vi "Align N Waveforms (continuous).vi"(4 "interpolation":bool=TRUE, 6 "FIR filter specifications":T1={"alias rejection (dB)"=120.0, "normalized bandwidth"=0.4536} {"normalized bandwidth" format="%.4f"; "alias rejection (dB)" format="%.2f"}, 7 "reset":bool, 8 "error in (no error)":errorcluster, 9 "interpolation mode":u16(ring)=1 items=["coerce", "linear", "spline", "FIR filter"], 11 "waveforms in":waveform(dbl)[](array[waveform])) -> (0 "error out":errorcluster, 3 "waveforms out":waveform(dbl)[](array[waveform]))   [LabVIEW 2020, in "NI_MAPro.lvlib"]
doc: "Performs element-wise alignment of waveforms and returns the aligned waveforms. The data types you wire to the waveform inputs determine the polymorphic instance to use."
uses:
  NI_MAPro.lvlib
  NI_MABase.lvlib
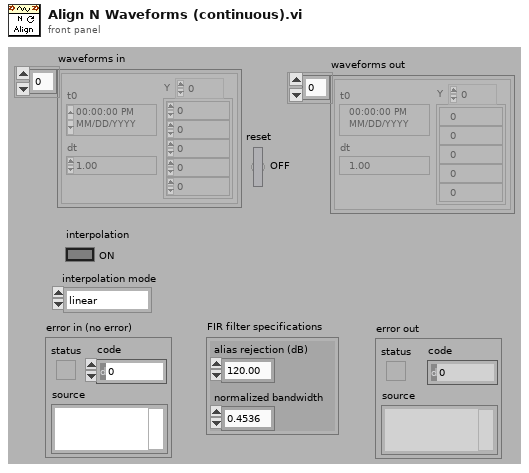
[diagram p1: front panel]
types:
  T1 = cluster{"alias rejection (dB)":dbl, "normalized bandwidth":dbl}
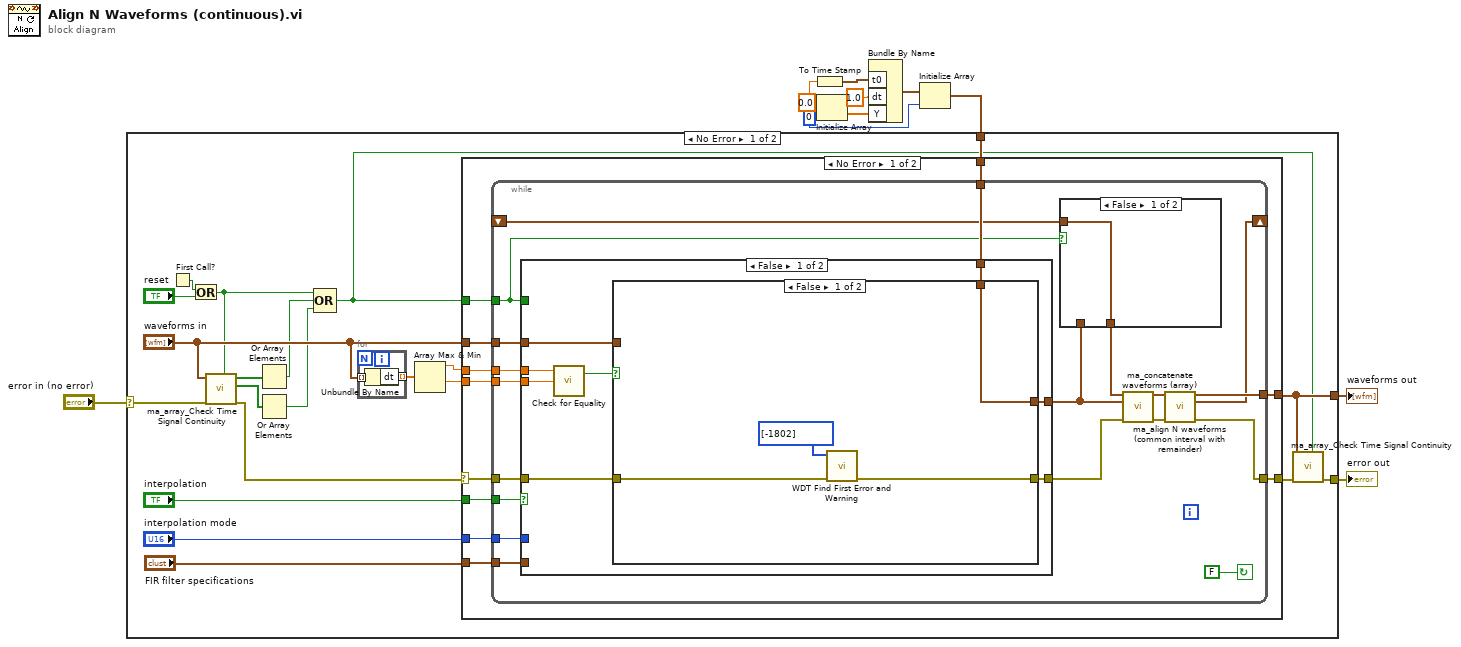
[diagram p0: block diagram]
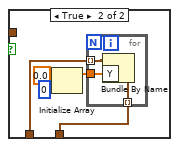
[diagram p2: hidden frame]
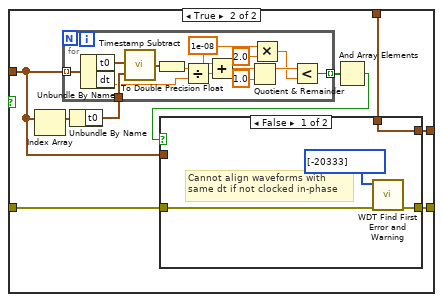
[diagram p3: hidden frame]
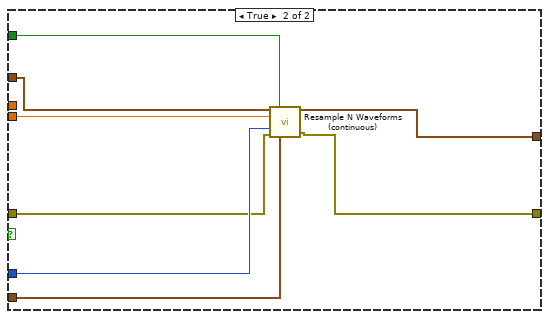
[diagram p5: hidden frame]
diagram:
  w4 = 0 ("dimension size")
  w7 = 0.0 ("element")
  n1 = To Time Stamp(1:w7) -> (0:w1:timestamp)
  n2 = Initialize Array(w7, w4) -> (w8:dbl[])
  n3 = Bundle By Name("t0"=w1, "dt"=1.0 ("element"), "Y"=w8) -> (w5:waveform(dbl))  [unwired: 1 in]
  n4 = Initialize Array(w5, w4) -> (w3:waveform(dbl)[])
  n5 = case shown="No Error" "error in (no error)" {
    selector: "error in (no error)" -> [w29 w125]
    tunnel: [w20 w125] -> w10
    tunnel: [w18 w124] -> w9
    tunnel: w3 -> [w25 w124]
    frame No Error {
      n6 = First Call?() -> (First Call?: T/F=w27:bool)
      n7 = Or(x=w27, y="reset") -> (x .or. y?=w17:bool)
      n8 = call "ma_array_Check Time Signal Continuity.vi"("Ignore input time stamp"=w17, "error in (no error)"=w29, "waveforms"="waveforms in") -> ("error out"=w14:errorcluster, "dt changed"=w13:bool[], "t0 changed"=w15:bool[])  [unwired: 5 in, 1 out]
      n9 = Or Array Elements(Boolean array=w15) -> (logical OR=w12:bool)
      n10 = Or Array Elements(Boolean array=w13) -> (logical OR=w11:bool)
      n11 = Compound Arithmetic op=OR(w17, w12, w11) -> (w16:bool)
      n12 = for {
        tunnel: "waveforms in" -> [w33] mode=indexing
        tunnel: [w32] -> w23 mode=indexing
        n13 = Unbundle By Name(w33) -> ("dt"=w32:dbl)
      }
      n14 = Array Max & Min(array=w23) -> (max value=w22:dbl, min value=w21:dbl)  [unwired: 2 out]
      n15 = case shown="No Error" w14 {
        selector: w14 -> [w39 w123]
        tunnel: "waveforms in" -> [w44 _]
        tunnel: w22 -> [w43 _]
        tunnel: w21 -> [w42 _]
        tunnel: [w38 w123] -> w19
        tunnel: [w41 w122] -> w18
        tunnel: w25 -> [w40 w122]
        tunnel: "interpolation mode" -> [w37 _]
        tunnel: "interpolation" -> [w36 _]
        tunnel: w16 -> [w35 _]
        tunnel: "FIR filter specifications" -> [w34 _]
        frame No Error {
          n16 = while {
            tunnel: w44 -> [w63]
            tunnel: w43 -> [w62]
            tunnel: w42 -> [w61]
            tunnel: [w53] -> w41
            tunnel: w40 -> [w60]
            tunnel: w39 -> [w59]
            tunnel: [w50] -> w38
            tunnel: w37 -> [w58]
            tunnel: w36 -> [w57]
            tunnel: w35 -> [w55]
            shift-right: [w47] -> _
            shift-left: _ -> [w45]
            tunnel: w34 -> [w48]
            stop <- FALSE continue-if-true
            n17 = case shown="False" w57 {
              tunnel: w63 -> [w80 w120]
              tunnel: w62 -> [w79 _]
              tunnel: w61 -> [w78 w118]
              tunnel: w60 -> [w76 _]
              tunnel: w59 -> [w75 w114]
              tunnel: [w74 w117] -> w52
              tunnel: w58 -> [_ w116]
              tunnel: w55 -> [_ w119]
              tunnel: w48 -> [_ w115]
              tunnel: [w73 w121] -> w46
              frame False {
                n18 = call "Check for Equality.vi"("n2"=w78, "n1"=w79) -> ("equal?"=w77:bool)  [unwired: 1 in, 1 out]
                n19 = case shown="False" w77 {
                  tunnel: w80 -> [_ w88]
                  tunnel: w76 -> [w81 w93]
                  tunnel: w75 -> [w84 w91]
                  tunnel: [w83 w92] -> w74
                  tunnel: [w81 w89] -> w73
                  frame False {
                    n20 = call "WDT Find First Error and Warning.vi"("error in (no error)"=w84, "Error Codes"=i32[] [-1802]) -> ("error out"=w83:errorcluster)  [unwired: 4 in, 1 out]
                  }
                  frame True {
                    n21 = Index Array(array=w88) -> (element=w87:waveform(dbl))  [unwired: 1 in]
                    n22 = Unbundle By Name(w87) -> ("t0"=w85:timestamp)
                    n23 = for {
                      tunnel: w88 -> [w107] mode=indexing
                      tunnel: w85 -> [w106]
                      tunnel: [w102] -> w90 mode=indexing
                      w99 = 1e-08
                      n24 = Unbundle By Name(w107) -> ("t0"=w96:timestamp, "dt"=w103:dbl)
                      n25 = call "Timestamp Subtract.vi"("y"=w106, "x"=w96) -> ("x - y"=w95:timestamp)
                      n26 = To Double Precision Float(number=w95) -> (double precision float=w94:dbl)
                      n27 = Divide(x=w94, y=w103) -> (x/y=w101:dbl)
                      n28 = Add(x=w99, y=w101) -> (x+y=w100:dbl)
                      n29 = Quotient & Remainder(x=w100, y=1.0) -> (x-y*floor(x/y)=w104:dbl)  [unwired: 1 out]
                      n30 = Multiply(x=w99, y=2.0) -> (x*y=w97:dbl)
                      n31 = Less?(x=w104, y=w97) -> (x < y?=w102:bool)
                    }
                    n32 = And Array Elements(Boolean array=w90) -> (logical AND=w86:bool)
                    n33 = case shown="False" w86 {
                      tunnel: [w108 w113] -> w92
                      tunnel: w91 -> [w109 w113]
                      tunnel: w93 -> [w111 _]
                      tunnel: w88 -> [_ w112]
                      tunnel: [w111 w112] -> w89
                      frame False {
                        # "Cannot align waveforms with\nsame dt if not clocked in-phase"
                        n34 = call "WDT Find First Error and Warning.vi"("error in (no error)"=w109, "Error Codes"=i32[] [-20333]) -> ("error out"=w108:errorcluster)  [unwired: 4 in, 1 out]
                      }
                      frame True {
                      }
                    }
                  }
                }
              }
              frame True {
                n35 = call "Resample N Waveforms (continuous).vi"("waveforms in"=w120, "reset"=w119, "dt"=w118, "interpolation mode"=w116, "error in (no error)"=w114, "FIR filter specifications"=w115) -> ("resampled waveforms out"=w121:waveform(dbl)[], "error out"=w117:errorcluster)  [unwired: 5 in, 3 out]
              }
            }
            n36 = case shown="False" w55 {
              tunnel: [w64 w69] -> w49
              tunnel: w46 -> [_ w65]
              tunnel: w45 -> [w64 _]
              frame False {
              }
              frame True {
                n37 = Initialize Array(0.0 ("element"), 0 ("dimension size")) -> (w66:dbl[])
                n38 = for {
                  tunnel: [w72] -> w69 mode=indexing
                  tunnel: w66 -> [w71]
                  tunnel: w65 -> [w70] mode=indexing
                  n39 = Bundle By Name(cluster=w70, "Y"=w71) -> (w72:waveform(dbl))
                }
              }
            }
            n40 = call "ma_concatenate waveforms (array).vi"("Waveforms A0 in"=w49, "Waveforms A1 in"=w46, "error in"=w52) -> ("Waveforms A out"=w54:waveform(dbl)[], "error out"=w51:errorcluster)  [unwired: 11 in]
            n41 = call "ma_align N waveforms (common interval with remainder).vi"("waveforms in"=w54, "error in"=w51) -> ("intersecting waveforms out"=w53:waveform(dbl)[], "remainder waveforms out"=w47:waveform(dbl)[], "error out"=w50:errorcluster)  [unwired: 11 in]
          }
        }
        frame Error {
        }
      }
      n42 = call "ma_array_Check Time Signal Continuity.vi"("Ignore input time stamp"=w16, "error in (no error)"=w19, "waveforms"=w18) -> ("error out"=w20:errorcluster)  [unwired: 5 in, 3 out]
    }
    frame Error {
    }
  }
  "error out" <- w10
  "waveforms out" <- w9
